vi "RP100SetSlew.vi"(2 "error in (no error)":errorcluster, 3 "Slew":dbl, 4 "Source":enum16{"1", "2", "Both"}(ring), 5 "VISA resource name":refnum<visa-resource-name>) -> (0 "error out":errorcluster, 1 "VISA resource name out":refnum<visa-resource-name>)   [LabVIEW 2019, in "RP100.lvlib"]
uses:
  RP100.lvlib
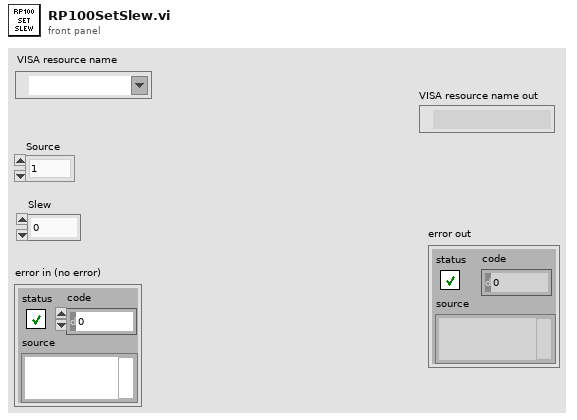
[diagram p1: front panel]
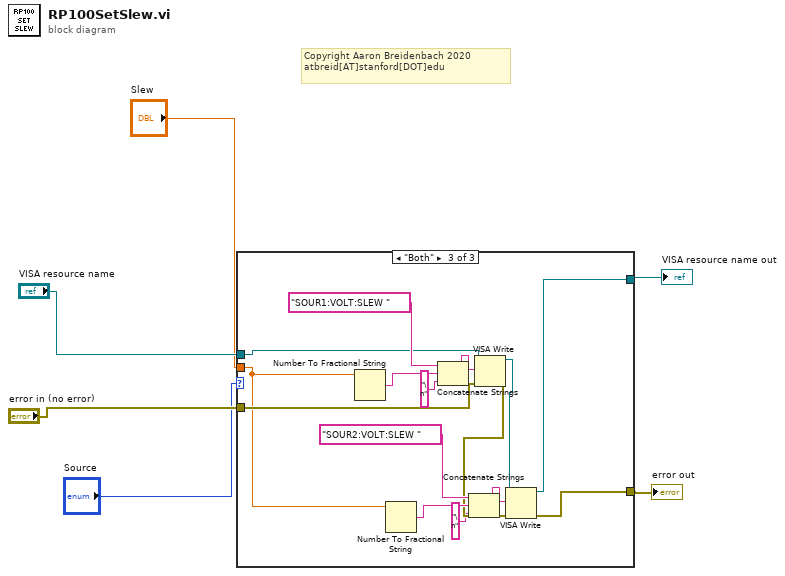
[diagram p0: block diagram]
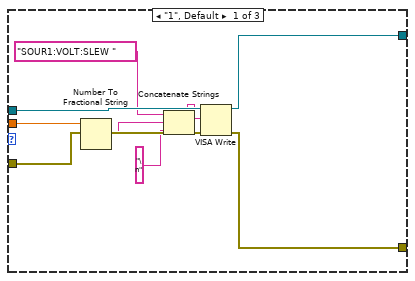
[diagram p2: hidden frame]
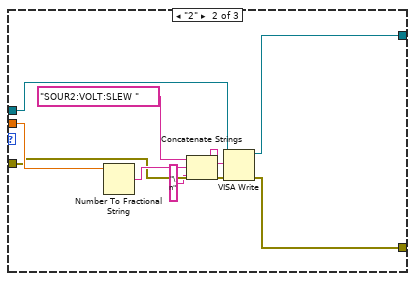
[diagram p3: hidden frame]
diagram:
  # "Copyright Aaron Breidenbach 2020\natbreid[AT]stanford[DOT]edu"
  n1 = case shown="\"Both\"" "Source" {
    tunnel: "VISA resource name" -> [w15 w18 w33]
    tunnel: "error in (no error)" -> [w14 w17 w30]
    tunnel: "Slew" -> [w10 w19 w27]
    tunnel: [w7 w20 w31] -> w5
    tunnel: [w8 w21 w32] -> w6
    frame "1", Default {
      n2 = Number To Fractional String(number=w10) -> (F-format string=w12:string)  [unwired: 3 in]
      n3 = Concatenate Strings("SOUR1:VOLT:SLEW " ("write buffer"), w12, "\n" ("string")) -> (w13:string)
      n4 = VISA Write(VISA resource name=w15, write buffer=w13, error in (no error)=w14) -> (VISA resource name out=w8:refnum<visa-resource-name>, error out=w7:errorcluster)  [unwired: 1 out]
    }
    frame "2" {
      n5 = Number To Fractional String(number=w19) -> (F-format string=w23:string)  [unwired: 3 in]
      n6 = Concatenate Strings("SOUR2:VOLT:SLEW " ("write buffer"), w23, "\n" ("string")) -> (w24:string)
      n7 = VISA Write(VISA resource name=w18, write buffer=w24, error in (no error)=w17) -> (VISA resource name out=w21:refnum<visa-resource-name>, error out=w20:errorcluster)  [unwired: 1 out]
    }
    frame "Both" {
      n8 = Number To Fractional String(number=w27) -> (F-format string=w38:string)  [unwired: 3 in]
      n9 = Number To Fractional String(number=w27) -> (F-format string=w35:string)  [unwired: 3 in]
      n10 = Concatenate Strings("SOUR1:VOLT:SLEW " ("write buffer"), w38, "\n" ("string")) -> (w39:string)
      n11 = Concatenate Strings("SOUR2:VOLT:SLEW " ("write buffer"), w35, "\n" ("string")) -> (w36:string)
      n12 = VISA Write(VISA resource name=w33, write buffer=w39, error in (no error)=w30) -> (VISA resource name out=w29:refnum<visa-resource-name>, error out=w28:errorcluster)  [unwired: 1 out]
      n13 = VISA Write(VISA resource name=w29, write buffer=w36, error in (no error)=w28) -> (VISA resource name out=w32:refnum<visa-resource-name>, error out=w31:errorcluster)  [unwired: 1 out]
    }
  }
  "error out" <- w5
  "VISA resource name out" <- w6
